vi "ClusterEscala.vi"() -> ()   [LabVIEW 2020]
panel:
  out "x*y 3":cluster{dbl, dbl, dbl}
  out "Cluster 5":T1 {"Gauge" scale=0.0..10.0; "Tank" scale=0.0..10.0; "Thermometer" scale=0.0..100.0}
  in  "Cluster 2":T2
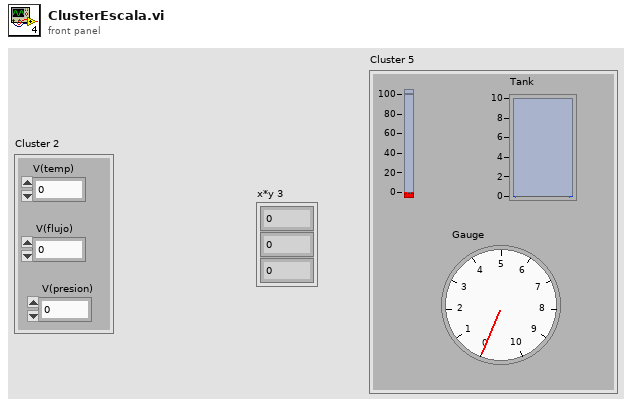
[diagram p1: front panel]
types:
  T1 = cluster{"Thermometer":dbl, "Tank":dbl, "Gauge":dbl}
  T2 = cluster{"V(temp)":dbl, " V(flujo)":dbl, " V(presion)":dbl}
  T3 = cluster{"°C/V":i32, "(1/seg)/V":i32, "(N/m^2)/V":i32}
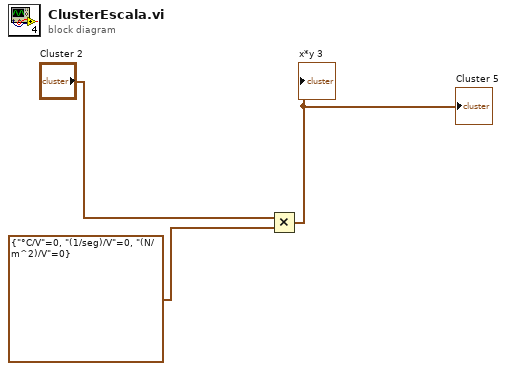
[diagram p0: block diagram]
diagram:
  n1 = Multiply(x="Cluster 2", y=T3 {"°C/V"=0, "(1/seg)/V"=0, "(N/m^2)/V"=0}) -> (x*y=→"Cluster 5" →"x*y 3":cluster{dbl, dbl, dbl})
